vi "ReceiveData.vi"(8 "错误输入（无错误）":errorcluster, 11 "连接ID":refnum<k5>) -> (0 "错误输出":errorcluster, 1 "head":string, 2 "dataOut":string, 3 "连接ID输出":refnum<k5>, 5 "字节数":u8)   [LabVIEW 2018]
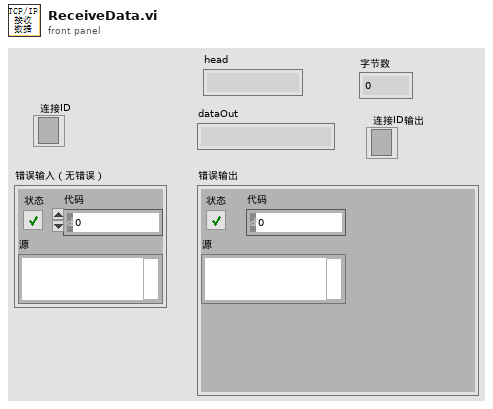
[diagram p1: front panel]
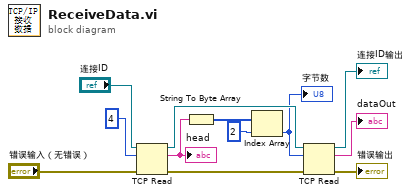
[diagram p0: block diagram]
diagram:
  n1 = TCP Read(connection ID="连接ID", bytes to read=u32 4 ("字节总数"), error in (no error)="错误输入（无错误）") -> (connection ID out=w2:refnum<k5>, data out=w6:string, error out=w5:errorcluster)  [unwired: 2 in]
  "head" <- w6
  n2 = String To Byte Array(string=w6) -> (unsigned byte array=w11:u8[])
  n3 = Index Array(array=w11, index=2 ("索引")) -> (element=w1:u8)
  "字节数" <- w1
  n4 = TCP Read(connection ID=w2, bytes to read=w1, error in (no error)=w5) -> (connection ID out=→"连接ID输出":refnum<k5>, data out=→"dataOut":string, error out=→"错误输出":errorcluster)  [unwired: 2 in]
